vi "absorbance.vi"(4 "Amax":dbl[](array[numeric])=[2.45484486000851, 2.54703589974001, 2.6248181855647315, 2.6325979848545886, 2.6312813855818904, 2.628142589680995, 2.684683817126539, 2.638589083292717, 2.6509870943834453, 2.7347190417019465, 2.7135745377720695, 2.699784844477403, 2.7726590342337167, 2.794975744051132, 2.7564375499733336, 2.8116554233288182, 2.776759279698738, 2.838370473760293, 2.73563003366452, 2.7702332534981964, 2.784132095185349, 2.7828594469279797, 2.769421639578743, 2.905407269252544, 2.8861070229313563, 2.87248259966074, 2.8647714610172246, 2.8675971086574776, 2.8773483057635643, 2.8971650641377704, 2.9204364065507584, 2.791901080009571, 2.815523956226929, 2.8348528754731213, 2.8445517263392732, 2.843083210487105, 2.8272787856106594, 2.800414616064902, 2.9214679730024424, 2.8818067615841425, 2.942305752895894, 2.9096410613382093, 2.885225481795713, 2.8747484587415375, 2.9518133303028518, 2.881144330134168, 2.8961402514420196, 2.9202167521932987, 2.9473650920544534, 2.8803333171261305, 2.91365493508662, 2.9495846635742646, 2.8225858214263693, 2.848447768581409, 2.866783392229962, 2.878475261456634, 2.8809849904867533, 2.878015973081706, 2.8680675427023616, 2.854767424335244, 2.8361848152550206, 2.8171149769762827, 2.9544161924977894, 2.9344782510304475, 2.915009163904051, 2.899174597304767, 2.884353483820743, 2.873715763680238, 2.9637023762207675, 2.9575881336286205, 2.9535755968832267, 2.9535755968832267, 2.953711380427555, 2.9591649816252223, 2.964137010754316, 2.9728135694324656, 2.880344758423387, 2.8903092168999485, 2.9000283014503423, 2.91184979649942, 2.9183973388437, 2.9286718078741467, 2.93407404933353, 2.9414219806233044, 2.9441267009381176, 2.946521039236374, 2.9454976356051223, 2.9150297621128076, 2.9166644645413973, 2.9700212658283656, 2.968623020956989, 2.9590695489626544, 2.9506082247842307, 2.9519778009651545, 2.9523467842241704, 2.9574343967439543, 2.938889318582866, 2.933588004143594, 2.9219568501428506, 2.934144306387223, 2.9945195122669848, 2.92096760458923, 2.9318233582278195, 2.9930745352785406, 2.9332943939715386, 2.9254668006915376, 2.9803124974029966, 2.9818543817806664, 2.9968792659013603, 2.9654274942714482, 2.9727950750437944, 2.975293915356206, 2.9927037056178887, 2.97455774485358, 2.9756890919776304, 2.994361151908001, 2.971405746462633, 2.9593753365758433, 2.9299392563278808, 2.9527246548916275, 2.9924823813741215, 2.9533923909543454, 2.96926677276395, 2.959461166467472, 2.9666016065702285, 2.971758130277843, 2.929674317948588, 2.9290508968483224, 2.9234719893019676, 2.911690158753861, 3.0095358766192177, 2.990525321584303, 2.969154884451621, 2.9767991749105738, 3.001897623714856, 2.99518750901127, 2.9497309647276015, 2.989200560793263, 2.9977004134241327, 3.0127275831330373, 3.01078275596756, 3.008301598140487, 2.96926677276395, 2.972711378088635, 2.954521815722125, 2.962871065533915, 2.9796844687345923, 2.977540705946535, 2.950003928420205, 2.959422545115349, 2.9875411414972066, 2.955475601200319, 3.008863648964221, 3.0039169907108327, 2.9746125405094737, 2.9888264070452757, 2.9931892517458647, 3.015208396693189, 2.995599659958957, 2.9981023361389605, 2.9786187003338025, 3.0098501611480364, 2.980748536076075, 3.0029604609825986, 3.0115535281955386, 3.0007636864410414, 3.00044232075289, 3.0025461731191667, 2.994167081740664, 3.001067052488375, 3.0014823202486713, 2.9995307084964926, 2.996905510695666, 3.0010150619278297, 3.0178427108836936, 2.9924563098165717, 3.008225324604515, 2.979448211387106, 3.0152419433409143, 3.0089317269355393, 3.009977509030925, 3.0101727032867784, 2.9971503856592268, 3.0189911789932635, 3.013199266923062, 2.9874785662617085, 2.9915361753000314, 2.979912410334717, 2.9953543477802915, 2.999539403689988, 2.929868315651473, 2.9863775563192263, 2.898659374409747, 2.882535921671527, 2.9767167043633824, 2.9282011955460288, 3.038628108711067, 3.035469763481282, 2.940546366552379, 2.934680210893603, 2.9643350711110794, 3.0060550865916427, 2.9191304138606142, 3.019041477298633, 3.0121958507472315, 2.9113813592906737, 2.8871214040631505, 2.8832752239392785, 3.0185253311833744, 3.0177255705412818, 2.94468003388131, 3.022320712201769, 2.950627688526532, 2.9949590994152313, 3.020700960343757, 2.988255647448529, 2.9740140184680937, 2.997010474015805, 3.017951068830742, 3.0133850177496853, 2.9918013562738675, 3.0189001284017296, 3.004329543601992, 3.00441553237823, 3.0214617850592993, 3.0145961346992247, 2.9551867964350085, 2.963438362958846, 2.938639790002001, 3.0005295163285988, 3.010045412636098, 3.022592901742472, 2.9373975165885065, 2.873366528789946, 3.006439941008353, 3.0020791941730787, 2.9862161985310416, 2.9373272821771135, 2.913972711550971, 2.862679866500334, 2.89291786783085, 3.0103508475425795, 2.924113291808946, 2.911806700090664, 2.9850310726899436, 3.0024075574018876, 2.993153516403604, 2.9962309536633835, 3.0225850683672997, 3.00552369267328, 3.021371251017942, 3.0096548218387076, 3.012094494533328, 2.9917486871310026, 3.0039342061737084, 2.979129356147615, 2.9577025628289, 2.9568208231866975, 2.9358396610470154, 3.023589884419411, 2.9945810812598945, 2.9750823941161197, 3.0084979728011207, 3.0189417063824706, 2.9547821468400484, 3.0101298529335008, 2.9878985414119605, 2.9699742647394665, 3.0008326124743703, 3.008804497562865, 3.0053173881057718, 2.9962401532444884, 3.0023129624054077, 3.0071671931470534, 2.9862067841425746, 3.0066367313605937, 2.9980499894286097, 2.9905519531637625, 2.9795028487874013, 3.0099006802767403, 2.9935155867056333, 3.008787474083965, 2.9820087674956324, 2.9919787909945836, 2.9992519353021754, 2.9736542320404085, 3.0102066411602326, 2.9905426322967146, 3.0154012545400386, 3.007858683843715, 3.0000260568872155, 2.9904454170459944, 3.0039600280885477, 2.952627796315486, 2.9630503170455986, 2.9989825600427946, 3.003744798538443, 3.0025461731191667, 3.0062344994387833, 2.994387549311506, 2.9896633526125176, 2.9558704714525326, 3.009773734490223, 3.0052830659884795, 2.9147973153812905, 2.9212805976238347, 2.8922282112077324, 2.870860201467077, 2.9317832153858596, 3.0100963333734874, 2.913962122747452, 2.832853018590731, 2.8431081419996067, 2.860709244517769, 2.799230238433963, 2.796282855735164] format="%.2f", 5 "Asample":dbl[](array[numeric])=[2.9, 2.9] format="%.2f") -> (1 "good data":bool[](array[boolean]))   [LabVIEW 2015]
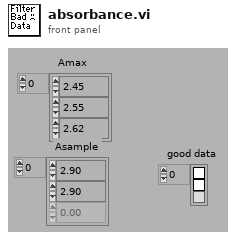
[diagram p1: front panel]
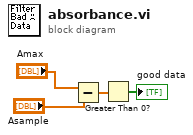
[diagram p0: block diagram]
diagram:
  n1 = Subtract(x="Amax", y="Asample") -> (x-y=w3:dbl[])
  n2 = Greater Than 0?(x=w3) -> (x > 0?=→"good data":bool[])
